vi "m1m3_logEvent_AppliedForces.vi"(8 "error in (no error)":errorcluster, 11 "logevent_AppliedForces_Ctl":T1) -> (0 "error out":errorcluster, 2 "function return":i32, 3 "logevent_AppliedForces_Ctl out":T1)   [LabVIEW 2016, in "SALLV_m1m3.lvlib"]
doc: "int m1m3_shm_logEvent_AppliedForcesLV(m1m3_logevent_AppliedForcesLV *logevent_AppliedForces_Ctl );"
uses:
  SALLV_m1m3.lvlib
  DataTypes/logevent_AppliedForces.ctl
  SALLV_m1m3/SALLV_m1m3.so
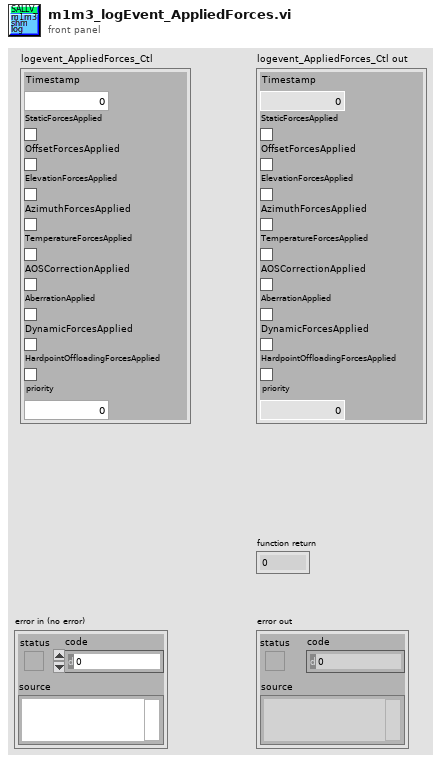
[diagram p1: front panel]
types:
  T1 = typedef "SALLV_m1m3.lvlib/logevent_AppliedForces.ctl" = cluster{"Timestamp":dbl, "StaticForcesApplied":bool, "OffsetForcesApplied":bool, "ElevationForcesApplied":bool, "AzimuthForcesApplied":bool, "TemperatureForcesApplied":bool, "AOSCorrectionApplied":bool, "AberrationApplied":bool, "DynamicForcesApplied":bool, "HardpointOffloadingForcesApplied":bool, "priority":i32}
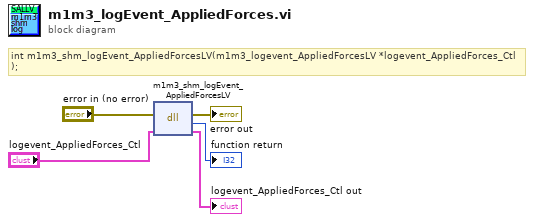
[diagram p0: block diagram]
diagram:
  # "int m1m3_shm_logEvent_AppliedForcesLV(m1m3_logevent_AppliedForcesLV *logevent_AppliedForces_Ctl );"
  n1 = dll-call lib="opt/CODE/SALLV_m1m3/SALLV_m1m3.*" fn="m1m3_shm_logEvent_AppliedForcesLV"(error in="error in (no error)", "logevent_AppliedForces_Ctl"="logevent_AppliedForces_Ctl") -> (error out=→"error out":errorcluster, →"function return":i32, "logevent_AppliedForces_Ctl"=→"logevent_AppliedForces_Ctl out":T1)  [unwired: 2 in, 1 out]
